vi "Check Error.vi"(0 "VISA Resource Name":refnum<visa-resource-name>, 5 "error in (no error)":errorcluster) -> (14 "dup VISA session":refnum<visa-resource-name>, 19 "error out":errorcluster)   [LabVIEW 2018, in "PNA-X.lvlib"]
uses:
  PNA-X.lvlib
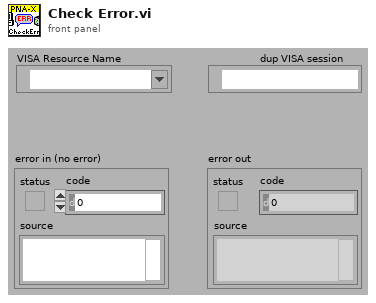
[diagram p1: front panel]
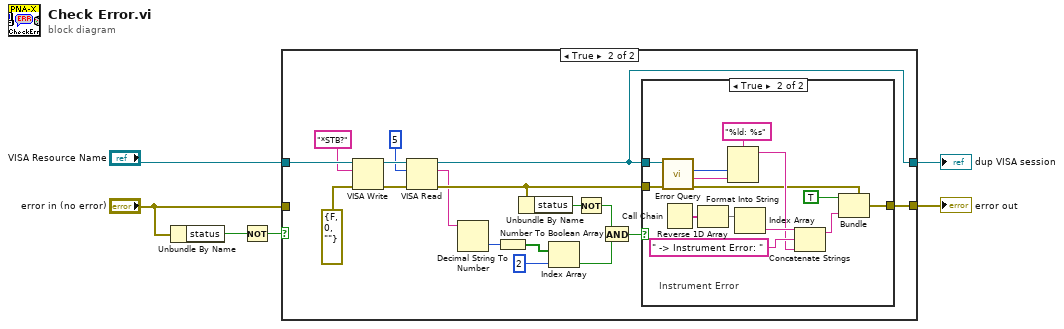
[diagram p0: block diagram]
diagram:
  n1 = Unbundle By Name("error in (no error)") -> ("status"=w2:bool)
  n2 = Not(x=w2) -> (.not. x?=w3:bool)
  n3 = case shown="True" w3 {
    tunnel: [w8 w23] -> w4
    tunnel: [w7 w17] -> w5
    tunnel: "VISA Resource Name" -> [w8 w16]
    tunnel: "error in (no error)" -> [w7 _]
    frame False {
      # "Communication error or error\nchecking turned off"
    }
    frame True {
      n4 = VISA Write(VISA resource name=w16, write buffer="*STB?" ("write buffer (\"\")"), error in (no error)=errorcluster {"status"=FALSE, "code"=0, "source"=""}) -> (VISA resource name out=w15:refnum<visa-resource-name>, error out=w14:errorcluster)  [unwired: 1 out]
      n5 = VISA Read(VISA resource name=w15, byte count=u32 5 ("byte count (0)"), error in (no error)=w14) -> (VISA resource name out=w23:refnum<visa-resource-name>, read buffer=w11:string, error out=w22:errorcluster)  [unwired: 1 out]
      n6 = Decimal String To Number(string=w11) -> (number=w10:i32)  [unwired: 2 in, 1 out]
      n7 = Number To Boolean Array(number=w10) -> (Boolean array=w25:bool[])
      n8 = Unbundle By Name(w22) -> ("status"=w21:bool)
      n9 = Index Array(array=w25, index=2) -> (element=w18:bool)
      n10 = Not(x=w21) -> (.not. x?=w19:bool)
      n11 = And(x=w19, y=w18) -> (x .and. y?=w20:bool)
      n12 = case shown="True" w20 {
        tunnel: w22 -> [w26 w31]
        tunnel: [w26 w39] -> w17
        tunnel: w23 -> [_ w30]
        frame False {
          # "No Error or IO Error"
        }
        frame True {
          # "Instrument Error"
          n13 = call "Error Query.vi"("error in (no error)"=w31, "VISA Resource Name"=w30) -> ("error out"=w29:errorcluster, "Error Message"=w28:string, "Error"=w27:i32)  [unwired: 4 in, 1 out]
          n14 = Call Chain() -> (call chain=w38:string[])
          n15 = Reverse 1D Array(array=w38) -> (reversed array=w37:string[])
          n16 = Format Into String(format string="%ld: %s", w27, w28) -> (resulting string=w32:string)  [unwired: 2 in, 1 out]
          n17 = Index Array(array=w37) -> (element=w34:string)  [unwired: 1 in]
          n18 = Concatenate Strings(w34, " -> Instrument Error: " ("string"), w32) -> (w35:string)
          n19 = Bundle(cluster=w29, "status"=TRUE, "source"=w35) -> (w39:errorcluster)  [unwired: 1 in]
        }
      }
    }
  }
  "error out" <- w5
  "dup VISA session" <- w4
